vi "DIGITAL WRITE TO READ.vi"(11 "DIGITAL WRITE in":bool[](array[boolean])) -> (3 "DIGITAL WRITE out":bool[](array[boolean]))   [LabVIEW 2019]
panel:
  in  "Reset allarmi":bool
  in  "Stop da operatore":bool
  in  "Allarme inv boost":bool
  in  "PRESSOSTATO ARIA":bool
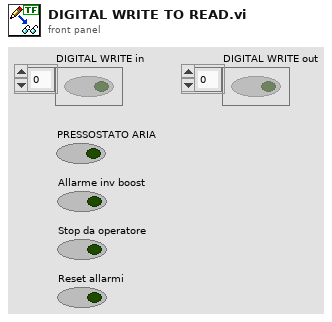
[diagram p1: front panel]
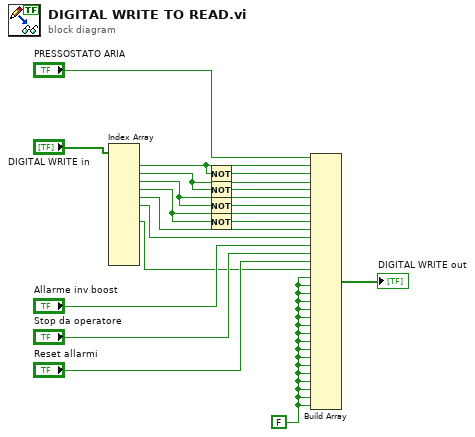
[diagram p0: block diagram]
diagram:
  w3 = FALSE ("element")
  n1 = Index Array(array="DIGITAL WRITE in") -> (element #1=w15:bool, element #2=w13:bool, element #3=w11:bool, element #4=w9:bool, element #5=w8:bool, element #6=w7:bool, element #8=w1:bool)  [unwired: 13 in, 6 out]
  n2 = Not(x=w15) -> (.not. x?=w16:bool)
  n3 = Not(x=w13) -> (.not. x?=w14:bool)
  n4 = Not(x=w11) -> (.not. x?=w12:bool)
  n5 = Not(x=w9) -> (.not. x?=w10:bool)
  n6 = Build Array("PRESSOSTATO ARIA", w15, w16, w13, w14, w11, w12, w9, w10, w8, w7, "Allarme inv boost", "Stop da operatore", "Reset allarmi", w1, w3, w3, w3, w3, w3, w3, w3, w3, w3, w3, w3, w3, w3, w3, w3, w3, w3) -> (→"DIGITAL WRITE out":bool[])
